vi "tearDown.vi"(8 "error in (no error)":errorcluster, 11 "reference in":refnum<class "testcase-csmhelper.lvclass">) -> (0 "error out":errorcluster, 3 "reference out":refnum<class "testcase-csmhelper.lvclass">)   [LabVIEW 2017, in "testcase-csmhelper.lvclass"]
doc: "tearDown runs after the test method has completed. Use this method to clean up any operations or references that were opened by setUp or the test method. Unit tests should be independent of other unit tests so this VI should ensure that the next test can run in a 'clean' test environment."
uses:
  testcase-csmhelper.lvclass
  testcase-csmhelper.lvclass/testcase-csmhelper.ctl
  src/user.lib/_NEVSTOP/Communicable State Machine(CSM)/Communicable State Machine.lvlib
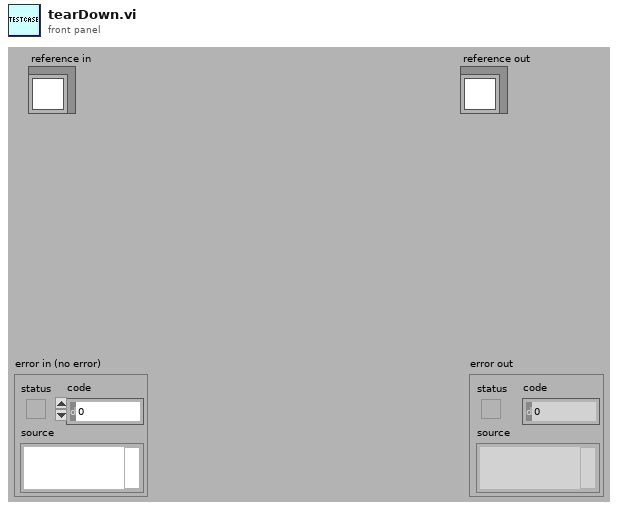
[diagram p1: front panel]
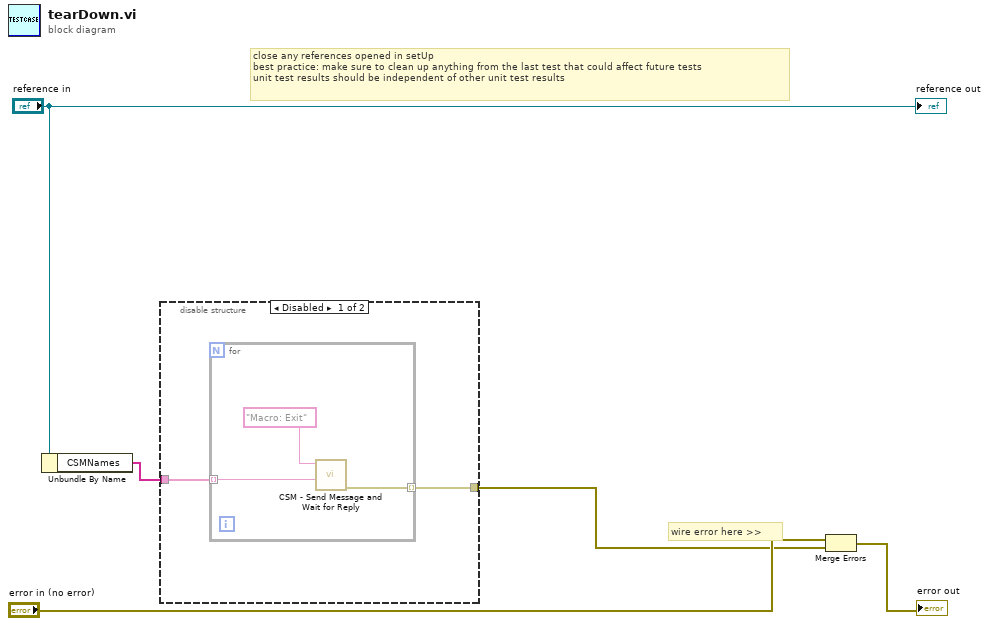
[diagram p0: block diagram]
diagram:
  # "wire error here >>"
  # "close any references opened in setUp\nbest practice: make sure to clean up anything from the last test that could affect future tests\nunit test results should be independent of other unit test results"
  n1 = Unbundle By Name("reference in") -> ("CSMNames"=w2:string[])
  n2 = disable-structure shown="Disabled" {
    disable-tunnel: w2 -> [w7 _]
    disable-tunnel: [w6 _] -> w1
    frame Disabled {
      n3 = for {
        tunnel: w7 -> [w9] mode=indexing
        tunnel: [w8] -> w6 mode=indexing
        n4 = call "CSM - Send Message and Wait for Reply.vi"("Target Module"=w9, "State"="Macro: Exit") -> ("error out"=w8:errorcluster)  [unwired: 7 in, 2 out]
      }
    }
    frame Enabled {
    }
  }
  n5 = Merge Errors("error in (no error)", w1) -> (→"error out":errorcluster)
  "reference out" <- "reference in"
